vi "End.vi"(8 "error in (no error)":errorcluster, 11 "S4ACS_GUI in":refnum<class "GuiderSetup.lvclass">) -> (0 "error out":errorcluster, 3 "S4ACS_GUI out":refnum<class "GuiderSetup.lvclass">)   [LabVIEW 2018, in "GuiderSetup.lvclass"]
uses:
  GuiderSetup.lvclass
  C:/Users/devstaff/sparc4/s4gui/Versao ZeroMQ REQ-REP/SPARC4_GUI -v1.0.0 - 20241216/S4GUI/S4GUI.lvclass
  S4GUI/S4GUI.lvclass/S4GUI.ctl
  Instrument/Instrument.lvclass
  AG/AG.lvclass
  PublisherGS/PublisherGS.lvclass
  S4GUI/S4GUI.lvclass
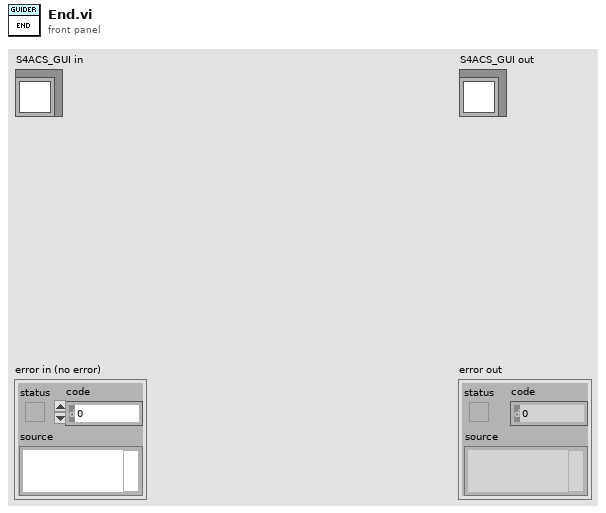
[diagram p1: front panel]
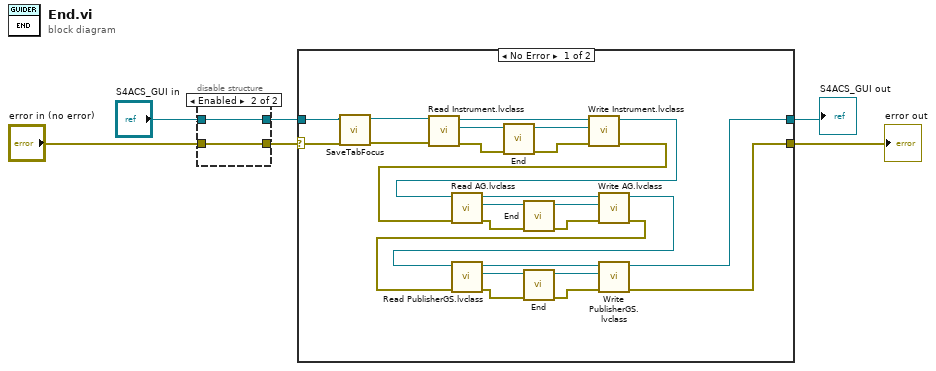
[diagram p0: block diagram]
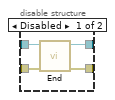
[diagram p2: hidden frame]
diagram:
  n1 = disable-structure shown="Enabled" {
    disable-tunnel: "error in (no error)" -> [w10 w11]
    disable-tunnel: "S4ACS_GUI in" -> [w9 w12]
    disable-tunnel: [w8 w11] -> w4
    disable-tunnel: [w7 w12] -> w3
    frame Disabled {
      n2 = call-parent "End.vi"("error in (no error)"=w10, "S4ACS_GUI in"=w9) -> ("error out"=w8:errorcluster, "S4ACS_GUI out"=w7:refnum<class "GuiderSetup.lvclass">)  [unwired: 8 in]
    }
    frame Enabled {
    }
  }
  n3 = case shown="No Error" w4 {
    selector: w4 -> [w23 w38]
    tunnel: w3 -> [w25 w39]
    tunnel: [w15 w38] -> w1
    tunnel: [w16 w39] -> w2
    frame No Error {
      n4 = call-dynamic "SaveTabFocus.vi"("error in (no error)"=w23, "GuiderSetup in"=w25) -> ("error out"=w22:errorcluster, "GuiderSetup out"=w24:refnum<class "GuiderSetup.lvclass">)  [unwired: 8 in]
      n5 = call "Read Instrument.lvclass.vi"("error in (no error)"=w22, "S4ACS_GUI in"=w24) -> ("error out"=w36:errorcluster, "Instrument.lvclass"=w37:refnum<class "Instrument.lvclass">, "S4ACS_GUI out"=w35:refnum<class "GuiderSetup.lvclass">)  [unwired: 7 in]
      n6 = call-dynamic "End.vi"("error in (no error)"=w36, "Server in"=w37) -> ("error out"=w33:errorcluster, "Server out"=w34:refnum<class "Instrument.lvclass">)  [unwired: 8 in]
      n7 = call "Write Instrument.lvclass.vi"("error in (no error)"=w33, "Instrument.lvclass"=w34, "S4ACS_GUI in"=w35) -> ("error out"=w28:errorcluster, "S4ACS_GUI out"=w27:refnum<class "GuiderSetup.lvclass">)  [unwired: 7 in]
      n8 = call-dynamic "Read AG.lvclass.vi"("error in (no error)"=w28, "GuiderSetup in"=w27) -> ("error out"=w30:errorcluster, "AG.lvclass"=w32:refnum<class "AG.lvclass">, "GuiderSetup out"=w26:refnum<class "GuiderSetup.lvclass">)  [unwired: 7 in]
      n9 = call-dynamic "End.vi"("error in (no error)"=w30, "Client in"=w32) -> ("error out"=w29:errorcluster, "Client out"=w31:refnum<class "AG.lvclass">)  [unwired: 8 in]
      n10 = call-dynamic "Write AG.lvclass.vi"("error in (no error)"=w29, "AG.lvclass"=w31, "GuiderSetup in"=w26) -> ("error out"=w19:errorcluster, "GuiderSetup out"=w18:refnum<class "GuiderSetup.lvclass">)  [unwired: 7 in]
      n11 = call-dynamic "Read PublisherGS.lvclass.vi"("error in (no error)"=w19, "GuiderSetup in"=w18) -> ("error out"=w21:errorcluster, "PublisherGS.lvclass"=w14:refnum<class "PublisherGS.lvclass">, "GuiderSetup out"=w17:refnum<class "GuiderSetup.lvclass">)  [unwired: 7 in]
      n12 = call-dynamic "End.vi"("error in (no error)"=w21, "PublisherGS in"=w14) -> ("error out"=w20:errorcluster, "PublisherGS out"=w13:refnum<class "PublisherGS.lvclass">)  [unwired: 8 in]
      n13 = call-dynamic "Write PublisherGS.lvclass.vi"("error in (no error)"=w20, "PublisherGS.lvclass"=w13, "GuiderSetup in"=w17) -> ("error out"=w15:errorcluster, "GuiderSetup out"=w16:refnum<class "GuiderSetup.lvclass">)  [unwired: 7 in]
    }
    frame Error {
    }
  }
  "error out" <- w1
  "S4ACS_GUI out" <- w2
